vi "Teleop.vi"(10 "Match Info":T1={"Autonomous Elapsed Seconds"=0.0, "TeleOp Elapsed Seconds"=0.0, "Disabled Elapsed Seconds"=0.0, "Visited Autonomous"=FALSE, "Visited TeleOp"=FALSE, "Visited Disabled"=FALSE, "Autonomous Settings"={"Autonomous Style"=enum."Independent", "VI Refnum"=refnum}}, 11 "Call Context":T2) -> ()   [LabVIEW 2016]
doc: "This VI is called for each TeleOp packet received from the DS where the robot is not disabled. It is often used to read from the joysticks and update I/O or to update setpoints for timed control loops. It should complete and return within 20 milliseconds or it may miss DS packets."
uses:
  <vilib>/Rock Robotics/WPI/DriverStation/WPI_DriverStationDerivedRobotMode.ctl
  <vilib>/Rock Robotics/WPI/DriverStation/WPI_DriverStationMatch Info.ctl
  <vilib>/Rock Robotics/WPI/Relay/WPI_RelayValue.ctl
  <vilib>/Rock Robotics/WPI/Solenoid/WPI_SolenoidValue.ctl
  <vilib>/Rock Robotics/WPI/Utilities/WPI_GetSetVariantRefNum.vi
  <vilib>/Rock Robotics/Network Tables/NT Write Boolean Array.vi
  <vilib>/Rock Robotics/Network Tables/NT Write Numeric Array.vi
  <vilib>/Rock Robotics/Network Tables/NT Write Number.vi
  <vilib>/Rock Robotics/WPI/Solenoid/WPI_SolenoidSetEnum.vi
  <vilib>/Rock Robotics/Network Tables/NT Read Boolean.vi
  <vilib>/Rock Robotics/Network Tables/NT Read Number.vi
panel:
  out "Sample Slider 0":dbl(slide) scale=0.0..5.0
  out "Sample Boolean 1":bool
  out "Sample Boolean 0":bool
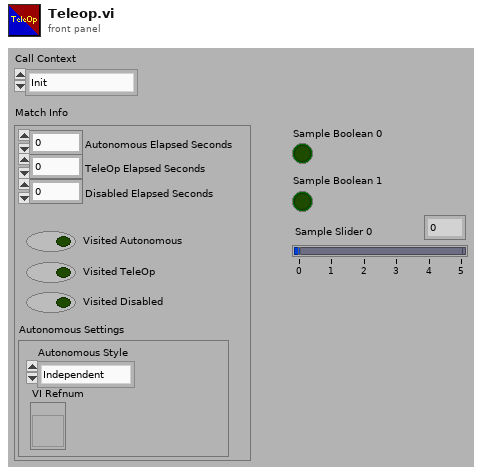
[diagram p1: front panel]
types:
  T1 = typedef "WPI_DriverStationMatch Info.ctl" = cluster{"Autonomous Elapsed Seconds":dbl, "TeleOp Elapsed Seconds":dbl, "Disabled Elapsed Seconds":dbl, "Visited Autonomous":bool, "Visited TeleOp":bool, "Visited Disabled":bool, "Autonomous Settings":cluster{"Autonomous Style":enum16{"Iterative", "Independent"}, "VI Refnum":refnum<vi>}}
  T2 = typedef "WPI_DriverStationDerivedRobotMode.ctl" = enum16{"Init", "Execute", "Stop"}
  T3 = typedef "WPI_SolenoidValue.ctl" = enum16{"Off", "On", "Forward", "Reverse"}
  T4 = typedef "WPI_RelayValue.ctl" = enum16{"Off", "On", "Forward", "Reverse"}
  T5 = typedef "WPI_JoystickDevRef.ctl" = cluster{"Device":T6}
  T6 = typedef "WPI_JoystickDeviceEnum.ctl" = enum16{"USB 0", "USB 1", "USB 2", "USB 3", "USB 4", "USB 5"}
  T7 = typedef "WPI_MotorControlDeviceRef.ctl" = cluster{"DeviceStatus":errorcluster, "Type":T8, "PWM":cluster{"PWM Channel":T9, "DeadBand":T10}, "CAN":cluster{"Device Number":u8, "SetOutput VI Ref":variant, "GetOutput VI Ref":variant, "Enable VI Ref":variant, "Disable VI Ref":variant, "Data":variant}, "Invert":bool}
  T8 = typedef "WPI_MotorControlType.ctl" = enum16{"PWM", "CAN"}
  T9 = typedef "FPGA_DIOPWMChannel.ctl" = enum8{"PWM 0", "PWM 1", "PWM 2", "PWM 3", "PWM 4", "PWM 5", "PWM 6", "PWM 7", "PWM 8", "PWM 9", "PWM MXP 0", "PWM MXP 1", "PWM MXP 2", "PWM MXP 3", "PWM MXP 4", "PWM MXP 5", "PWM MXP 6", "PWM MXP 7", "PWM MXP 8", "PWM MXP 9", "Invalid"}
  T10 = typedef "WPI_PWMDeadband.ctl" = cluster{"Name":string, "maxPositivePwm":i32, "minPositivePwm":i32, "centerPwm":i32, "maxNegativePwm":i32, "minNegativePwm":i32, "angularRange":u16}
  T11 = typedef "WPI_SolenoidDevRef.ctl" = cluster{"DevStatus":errorcluster, "Pneumatics Control Module":u8, "Forward Solenoid Channel":T12, "Reverse Solenoid Channel":T12}
  T12 = typedef "WPI_SolenoidChannel.ctl" = enum8{"Solenoid 0", "Solenoid 1", "Solenoid 2", "Solenoid 3", "Solenoid 4", "Solenoid 5", "Solenoid 6", "Solenoid 7", "Invalid"}
  T13 = typedef "WPI_RelayDevRef.ctl" = cluster{"DevStatus":errorcluster, "Relay Channel":T14, "Relay Direction":T15}
  T14 = typedef "FPGA_DIORelayChannel.ctl" = enum8{"Relay 0", "Relay 1", "Relay 2", "Relay 3", "Invalid"}
  T15 = typedef "WPI_RelayDirection.ctl" = enum16{"Both directions", "Forward only", "Reverse only"}
  T16 = typedef "WPI_RobotDriveDevRef.ctl" = cluster{"DevStatus":errorcluster, "Motors[]":T7[], "Square Inputs":bool, "Max Output":dbl}
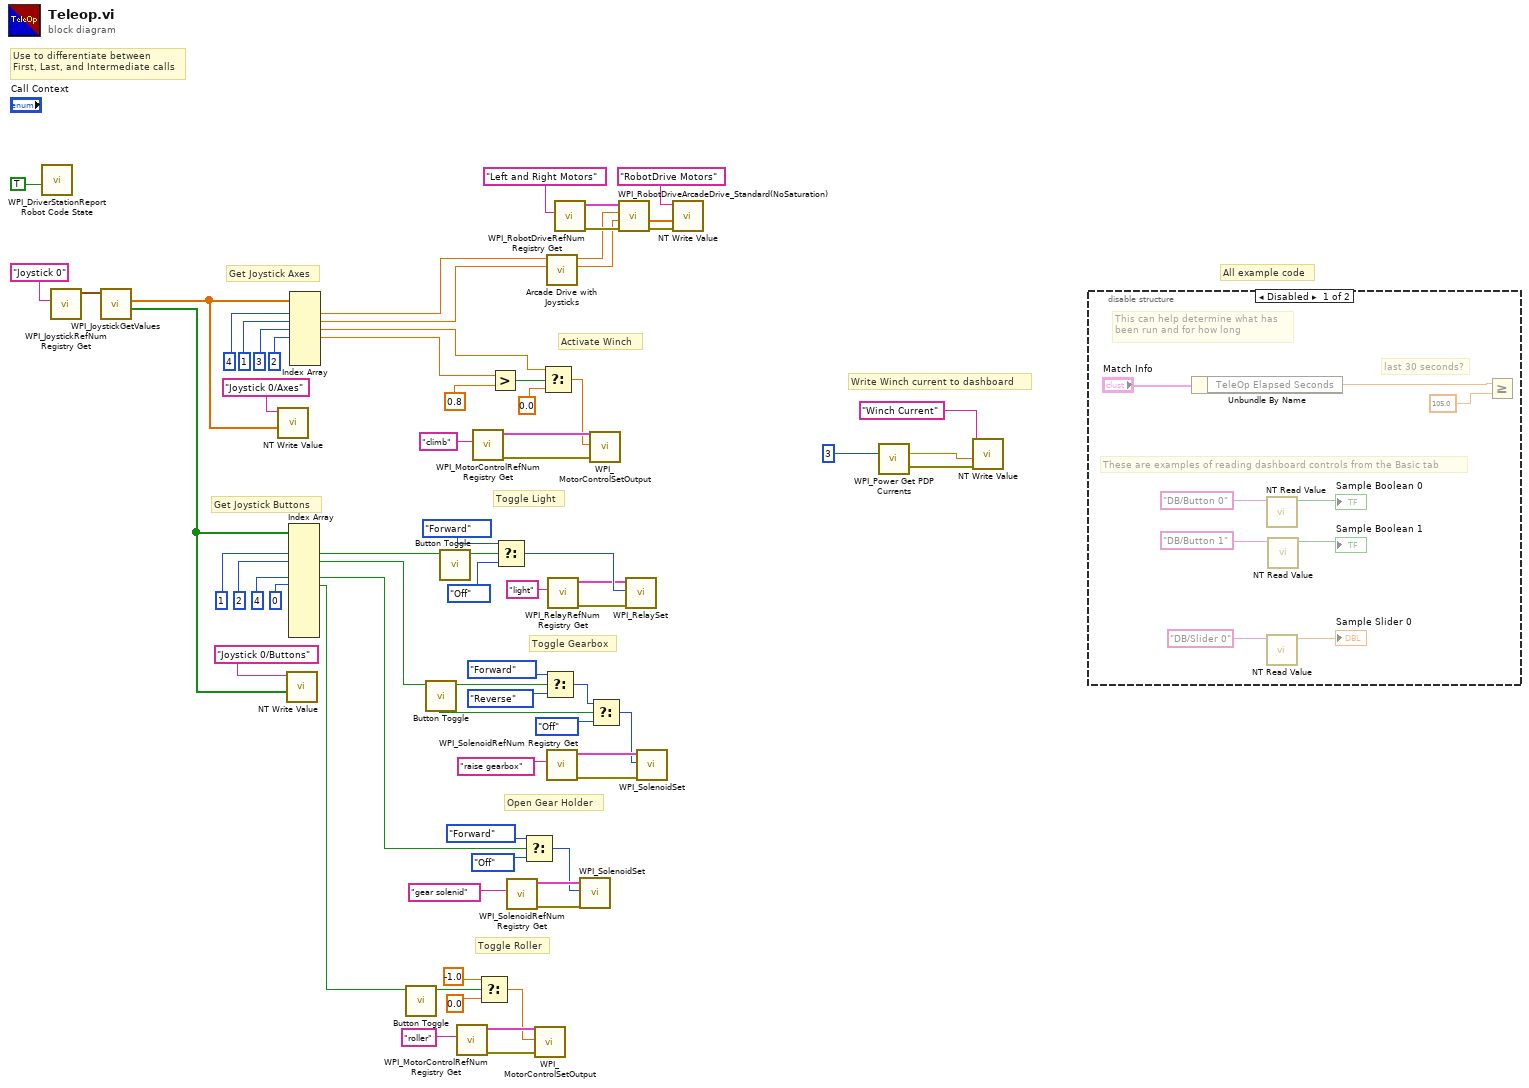
[diagram p0: block diagram]
diagram:
  # "Write Winch current to dashboard"
  # "Open Gear Holder"
  # "Get Joystick Buttons"
  # "Activate Winch"
  # "Get Joystick Axes"
  # "All example code"
  # "Toggle Gearbox"
  # "Toggle Roller"
  # "Toggle Light"
  # "Use to differentiate between\nFirst, Last, and Intermediate calls"
  n1 = call <vilib>:"WPI_DriverStationReport Robot Code State.vi"("TeleOp"=TRUE ("Autonomous")) -> ()  [unwired: 10 in, 1 out]
  n2 = call <vilib>:"WPI_JoystickRefNum Registry Get.vi"("refnum name"="Joystick 0") -> ("JoystickDevRef"=w69:T5)  [unwired: 1 in, 9 out]
  n3 = call <vilib>:"WPI_JoystickGetValues.vi"("JoystickDevRef"=w69) -> ("Buttons"=w60:bool[], "Axes"=w65:dbl[])  [unwired: 6 in, 3 out]
  n4 = call-poly <vilib>:"NT Write Value.vi"("Numeric Array"=w65, "Name"="Joystick 0/Axes") -> ()  [unwired: 9 in, 1 out]
  n5 = call-poly <vilib>:"NT Write Value.vi"("Boolean Array"=w60, "Name"="Joystick 0/Buttons") -> ()  [unwired: 9 in, 1 out]
  n6 = Index Array(array=w60, index #2=1 ("index"), index #3=2 ("index"), index #5=4 ("index"), index #6=0 ("index")) -> (element #2=w51:bool, element #3=w26:bool, element #5=w28:bool, element #6=w11:bool)  [unwired: 8 in, 8 out]
  n7 = Index Array(array=w65, index #1=4 ("index"), index #2=1 ("index"), index #3=3 ("index"), index #4=2 ("index")) -> (element #1=w6:dbl, element #2=w5:dbl, element #3=w36:dbl, element #4=w38:dbl)  [unwired: 3 in, 3 out]
  n8 = call "Button Toggle.vi"("Button In"=w11) -> ("Toggle Out"=w12:bool)  [unwired: 9 in, 1 out]
  n9 = call "Button Toggle.vi"("Button In"=w26) -> ("One-Shot Out"=w23:bool, "Toggle Out"=w22:bool)  [unwired: 9 in]
  n10 = call "Button Toggle.vi"("Button In"=w51) -> ("Toggle Out"=w50:bool)  [unwired: 9 in, 1 out]
  n11 = call <vilib>:"WPI_MotorControlRefNum Registry Get.vi"("refnum name"="roller") -> ("error out"=w13:errorcluster, "MotorControlDevRef"=w14:T7)  [unwired: 9 in]
  n12 = call <vilib>:"WPI_MotorControlRefNum Registry Get.vi"("refnum name"="climb") -> ("error out"=w54:errorcluster, "MotorControlDevRef"=w55:T7)  [unwired: 9 in]
  n13 = Select(t=-1.0, s=w12, f=0.0) -> (s? t:f=w7:dbl)
  n14 = Greater?(x=w38, y=0.8) -> (0:w4:bool)
  n15 = Select(t=WPI_RelayValue."Forward" ("RelayValue"), s=w50, f=WPI_RelayValue."Off" ("RelayValue")) -> (s? t:f=w47:T4)
  n16 = call <vilib>:"WPI_SolenoidRefNum Registry Get.vi"("refnum name"="gear solenid") -> ("error out"=w57:errorcluster, "SolenoidDevRef"=w58:T11)  [unwired: 9 in]
  n17 = Select(t=WPI_SolenoidValue."Forward", s=w28, f=WPI_SolenoidValue."Off" ("Value")) -> (s? t:f=w27:T3)
  n18 = call <vilib>:"WPI_MotorControlSetOutput.vi"("error in (no error)"=w13, "Output"=w7, "MotorControlDevRef"=w14) -> ()  [unwired: 6 in, 3 out]
  n19 = Select(t=w36, s=w4, f=0.0) -> (s? t:f=w3:dbl)
  n20 = Select(t=WPI_SolenoidValue."Forward" ("Value"), s=w22, f=WPI_SolenoidValue."Reverse" ("Value")) -> (s? t:f=w20:T3)
  n21 = call "Arcade Drive with Joysticks.vi"("Y Axis"=w5, "X Axis"=w6) -> ("Speed"=w1:dbl, "Turn"=w2:dbl)  [unwired: 8 in]
  n22 = call <vilib>:"WPI_SolenoidRefNum Registry Get.vi"("refnum name"="raise gearbox") -> ("error out"=w43:errorcluster, "SolenoidDevRef"=w42:T11)  [unwired: 9 in]
  n23 = call <vilib>:"WPI_RelayRefNum Registry Get.vi"("refnum name"="light") -> ("error out"=w45:errorcluster, "RelayDevRef"=w46:T13)  [unwired: 9 in]
  n24 = call <vilib>:"WPI_RobotDriveRefNum Registry Get.vi"("refnum name"="Left and Right Motors") -> ("error out"=w33:errorcluster, "RobotDriveDevRef"=w71:T16)  [unwired: 1 in, 8 out]
  n25 = call-poly <vilib>:"WPI_SolenoidSet.vi"("error in (no error)"=w57, "Value"=w27, "SolenoidDevRef"=w58) -> ()  [unwired: 7 in, 2 out]
  n26 = call <vilib>:"WPI_MotorControlSetOutput.vi"("error in (no error)"=w54, "Output"=w3, "MotorControlDevRef"=w55) -> ()  [unwired: 6 in, 3 out]
  n27 = Select(t=w20, s=w23, f=WPI_SolenoidValue."Off" ("Value")) -> (s? t:f=w41:T3)
  n28 = call <vilib>:"WPI_RobotDriveArcadeDrive_Standard(NoSaturation).vi"("error in (no error)"=w33, "Y axis value"=w1, "X axis value"=w2, "RobotDriveDevRef"=w71) -> ("error out"=w34:errorcluster, "Motor Values"=w64:dbl[])  [unwired: 6 out]
  n29 = call <vilib>:"WPI_RelaySet.vi"("error in (no error)"=w45, "RelayValue"=w47, "RelayDevRef"=w46) -> ()  [unwired: 7 in, 2 out]
  n30 = call-poly <vilib>:"WPI_SolenoidSet.vi"("error in (no error)"=w43, "Value"=w41, "SolenoidDevRef"=w42) -> ()  [unwired: 7 in, 2 out]
  n31 = call-poly <vilib>:"NT Write Value.vi"("error in"=w34, "Numeric Array"=w64, "Name"="RobotDrive Motors") -> ()  [unwired: 8 in, 1 out]
  n32 = call <vilib>:"WPI_Power Get PDP Currents.vi"("PDP Channel"=3) -> ("current (A)"=w16:dbl, "error out"=w18:errorcluster)  [unwired: 12 in, 1 out]
  n33 = call-poly <vilib>:"NT Write Value.vi"("error in"=w18, "Numeric"=w16, "Name"="Winch Current") -> ()  [unwired: 8 in, 1 out]
  n34 = disable-structure shown="Disabled" {
    frame Disabled {
      # "last 30 seconds?"
      # "These are examples of reading dashboard controls from the Basic tab"
      # "This can help determine what has\nbeen run and for how long"
      n35 = Unbundle By Name("Match Info") -> ("TeleOp Elapsed Seconds"=w74:dbl)
      n36 = call-poly <vilib>:"NT Read Value.vi"("Name"="DB/Button 0" ("refnum name")) -> ("Boolean"=→"Sample Boolean 0":bool)  [unwired: 9 in, 1 out]
      n37 = call-poly <vilib>:"NT Read Value.vi"("Name"="DB/Slider 0" ("refnum name")) -> ("Numeric"=→"Sample Slider 0":dbl)  [unwired: 9 in, 1 out]
      n38 = call-poly <vilib>:"NT Read Value.vi"("Name"="DB/Button 1" ("refnum name")) -> ("Boolean"=→"Sample Boolean 1":bool)  [unwired: 9 in, 1 out]
      n39 = Greater Or Equal?(x=w74, y=105.0) -> ()  [unwired: 1 out]
    }
    frame Enabled {
    }
  }
